vi "niDTS Comm String Wait For ACK.vi"(8 "error in (no error)":errorcluster, 9 "Timeout (ms)":i32=1000, 10 "ACK":string, 11 "Comm String Handle":T1) -> (0 "error out":errorcluster, 1 "Sucess":bool, 2 "Response":string, 3 "Comm String Handle Out":T1)   [LabVIEW 2014, in "niDTS CommLib.lvlib"]
uses:
  niDTS CommLib.lvlib
  Includes/niDTS Comm String INC Handle.ctl
  Objects/String_class/niDTS Comm String.lvclass
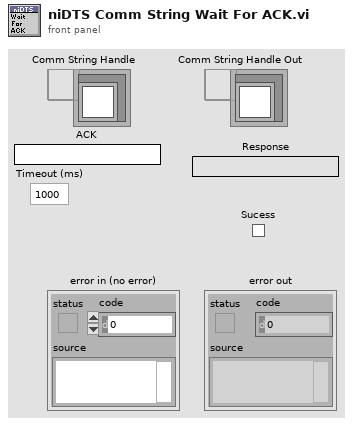
[diagram p1: front panel]
types:
  T1 = typedef "niDTS CommLib.lvlib/niDTS Comm String INC Handle.ctl" = refnum<data-value>
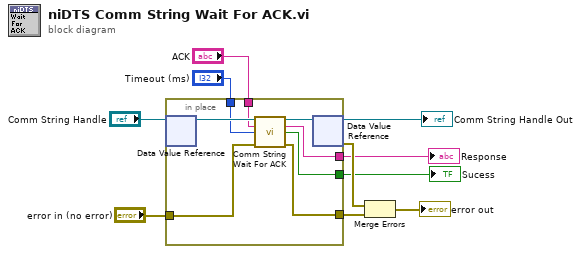
[diagram p0: block diagram]
diagram:
  n1 = in-place {
    in-place-border: "error in (no error)" -> [w17]
    in-place-border: "Timeout (ms)" -> [w16]
    in-place-border: "ACK" -> [w15]
    in-place-border: [w13] -> w6
    in-place-border: [w12] -> w2
    in-place-border: [w11] -> w1
    n2 = in-place-dvr #1("Comm String Handle") -> (w18:refnum<class "niDTS Comm String.lvclass">)  [unwired: 1 out]
    n3 = call-dynamic "Comm String Wait For ACK.vi"("niDTS Comm String in"=w18, "ACK"=w15, "Timeout (ms)"=w16, "error in (no error)"=w17) -> ("niDTS Comm String out"=w14:refnum<class "niDTS Comm String.lvclass">, "Response"=w12:string, "Sucess"=w11:bool, "error out"=w13:errorcluster)  [unwired: 8 in]
    n4 = in-place-dvr #1(w14) -> (→"Comm String Handle Out":T1, w5:errorcluster)
  }
  "Response" <- w2
  "Sucess" <- w1
  n5 = Merge Errors(w5, w6) -> (→"error out":errorcluster)
